vi "GetNamepatInfoByIndex.vi"(10 "Namepath Index":i32, 11 "NamePath":string[](array[string])) -> (0 "At path end":bool, 1 "Namepart found?":bool, 3 "Name":string)   [LabVIEW 2017]
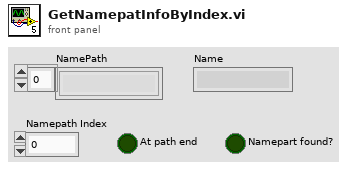
[diagram p1: front panel]
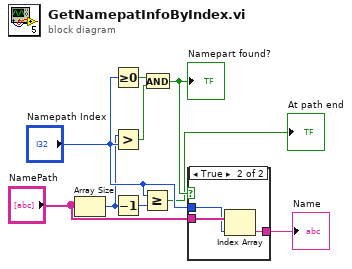
[diagram p0: block diagram]
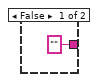
[diagram p2: hidden frame]
diagram:
  n1 = Array Size(array="NamePath") -> (size(s)=w1:i32)
  n2 = Greater Or Equal To 0?(x="Namepath Index") -> (x >= 0?=w6:bool)
  n3 = Greater?(x=w1, y="Namepath Index") -> (0:w7:bool)
  n4 = Decrement(x=w1) -> (x-1=w2:i32)
  n5 = Greater Or Equal?(x="Namepath Index", y=w2) -> (x >= y?=→"At path end":bool)
  n6 = And(x=w6, y=w7) -> (x .and. y?=w5:bool)
  "Namepart found?" <- w5
  n7 = case shown="True" w5 {
    tunnel: "NamePath" -> [_ w13]
    tunnel: "Namepath Index" -> [_ w12]
    tunnel: ["" ("Name") w11] -> w9
    frame False {
    }
    frame True {
      n8 = Index Array(array=w13, index=w12) -> (element=w11:string)
    }
  }
  "Name" <- w9
